vi "Service Close.vi"(8 "error in (no error)":errorcluster, 11 "Service Refs Cluster":T1) -> (0 "error out":errorcluster)   [LabVIEW 2010, in "CAN Log Transfer and Convert.lvlib"]
uses:
  CAN Log Transfer and Convert.lvlib
  Service Ref Cluster.ctl
  Queue Typedef.ctl
  <vilib>/NI Veristand/Execution/Workspace/WorkspaceAPI.ctl
  NationalInstruments.VeriStand.ClientAPI
  <vilib>/NI Veristand/Execution/Stimulus/StimulusAPI.ctl
  <vilib>/NI Veristand/Execution/Workspace/SystemStateRegEventRef.ctl
  <vilib>/NI Veristand/Execution/Workspace/SystemStateEventRef.ctl
  CAN Sysdef Data.ctl
  <vilib>/NI Veristand/Execution/Workspace/NI_VS Workspace ExecutionAPI.lvlib
  <vilib>/NI Veristand/Execution/Stimulus/NI_VS Stimulus ExecutionAPI.lvlib
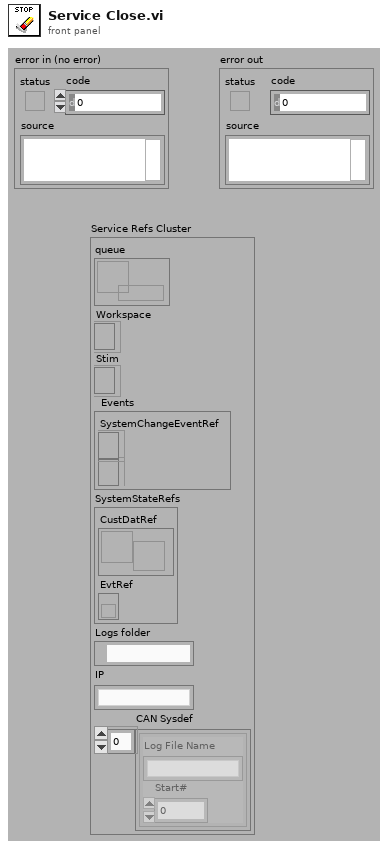
[diagram p1: front panel]
types:
  T1 = typedef "CAN Log Transfer and Convert.lvlib/Service Ref Cluster.ctl" = cluster{"queue":refnum<queue>, "Workspace":T2, "Stim":T3, "Events":cluster{"SystemChangeEventRef":T4, "NIVS.Workspace Event":refnum<event-registration>}, "SystemStateRefs":T5, "Logs folder":path, "IP":string, "CAN Sysdef":T6[]}
  T2 = typedef "NI_VS Workspace ExecutionAPI.lvlib/WorkspaceAPI.ctl" = refnum<k24>
  T3 = typedef "NI_VS Stimulus ExecutionAPI.lvlib/StimulusAPI.ctl" = refnum<k24>
  T4 = typedef "NI_VS Workspace ExecutionAPI.lvlib/SystemStateRegEventRef.ctl" = refnum<event-registration>
  T5 = typedef "NI_VS Workspace ExecutionAPI.lvlib/SystemStateEventRef.ctl" = cluster{"CustDatRef":refnum<user-event>, "EvtRef":refnum<k27>}
  T6 = typedef "CAN Log Transfer and Convert.lvlib/CAN Sysdef Data.ctl" = cluster{"Log File Name":string, "Start#":u16}
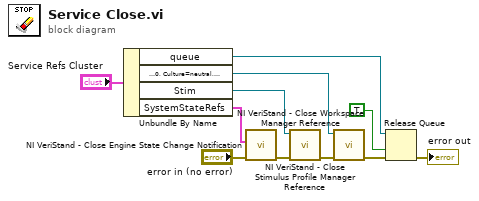
[diagram p0: block diagram]
diagram:
  n1 = Unbundle By Name("Service Refs Cluster") -> ("queue"=w9:refnum<queue>, "Workspace"=w8:T2, "Stim"=w7:T3, "SystemStateRefs"=w6:T5)
  n2 = call <vilib>:"NI VeriStand - Close Engine State Change Notification.vi"("error in (no error)"="error in (no error)", "SystemStateRefs"=w6) -> ("error out"=w5:errorcluster)  [unwired: 9 in]
  n3 = call <vilib>:"NI VeriStand - Close Stimulus Profile Manager Reference.vi"("error in (no error)"=w5, "StimulusProfileManager"=w7) -> ("error out"=w4:errorcluster)  [unwired: 9 in]
  n4 = call <vilib>:"NI VeriStand - Close Workspace Manager Reference.vi"("error in (no error)"=w4, "WorkspaceManager"=w8) -> ("error out"=w3:errorcluster)  [unwired: 9 in]
  n5 = Release Queue(queue=w9, force destroy? (F)=TRUE, error in (no error)=w3) -> (error out=→"error out":errorcluster)  [unwired: 2 out]
